vi "GoToCoordinate.vi"(0 "Target X":dbl=nan, 1 "Speed Multiplier (1)":dbl=1.0 format="%#_13g", 2 "Face PID Gains":T1={"proportional gain (Kc)"=0.275, "integral time (Ti, min)"=0.0, "derivative time (Td, min)"=0.006} {"derivative time (Td, min)" format="%.3f"; "integral time (Ti, min)" format="%.3f"; "proportional gain (Kc)" format="%.3f"}, 3 "Distance PID gains":T1={"proportional gain (Kc)"=0.0125, "integral time (Ti, min)"=0.0, "derivative time (Td, min)"=0.00225} {"derivative time (Td, min)" format="%_5g"; "integral time (Ti, min)" format="%_5g"; "proportional gain (Kc)" format="%_5g"}, 5 "Target Y":dbl=nan, 7 "Target Angle (rad)":dbl(knob)=nan scale=3.1416..-3.1416, 11 "error in (no error)":errorcluster, 12 "Position Tolerance":dbl, 14 "Angle Tolerance":dbl) -> (6 "Finished":bool, 15 "error out":errorcluster)   [LabVIEW 2015, in "Team900SwerveDrive.lvlib"]
uses:
  Team900SwerveDrive.lvlib
  SwerveGlobalData.vi
  <vilib>/addons/control/pid/NI_PID_pid.lvlib
  SwerveDriveFace.vi
  <vilib>/addons/control/pid/pid.llb/PID (DBL).vi
panel:
  out "Waveform Chart":cluster{"setpoint":dbl, dbl}(graph)
  # "Run this inside a while loop to autonomously move\nthe robot to target coordinates; the finished output\nwill become true when the robot is within tolerance\nof the target position (use this to terminate the \nwhile loop). If one or more elements of the target\ncoordinates are not wired, it will maintain the last\ninput position for that element\n\nPosition and Angle tolerance have no defaul values;\nall other terminals do not need to be wired."
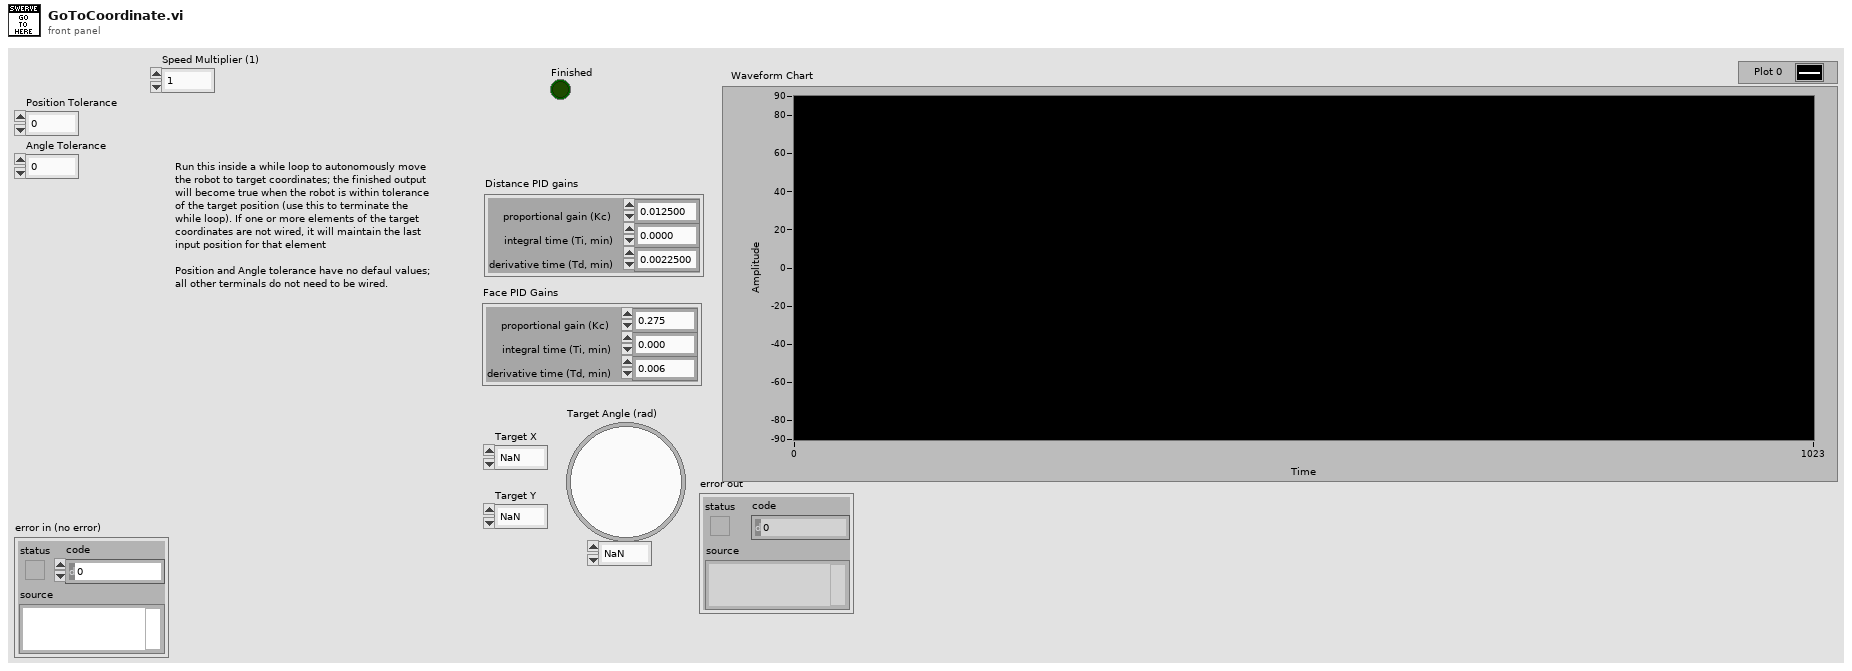
[diagram p1: front panel]
types:
  T1 = cluster{"proportional gain (Kc)":dbl, "integral time (Ti, min)":dbl, "derivative time (Td, min)":dbl}
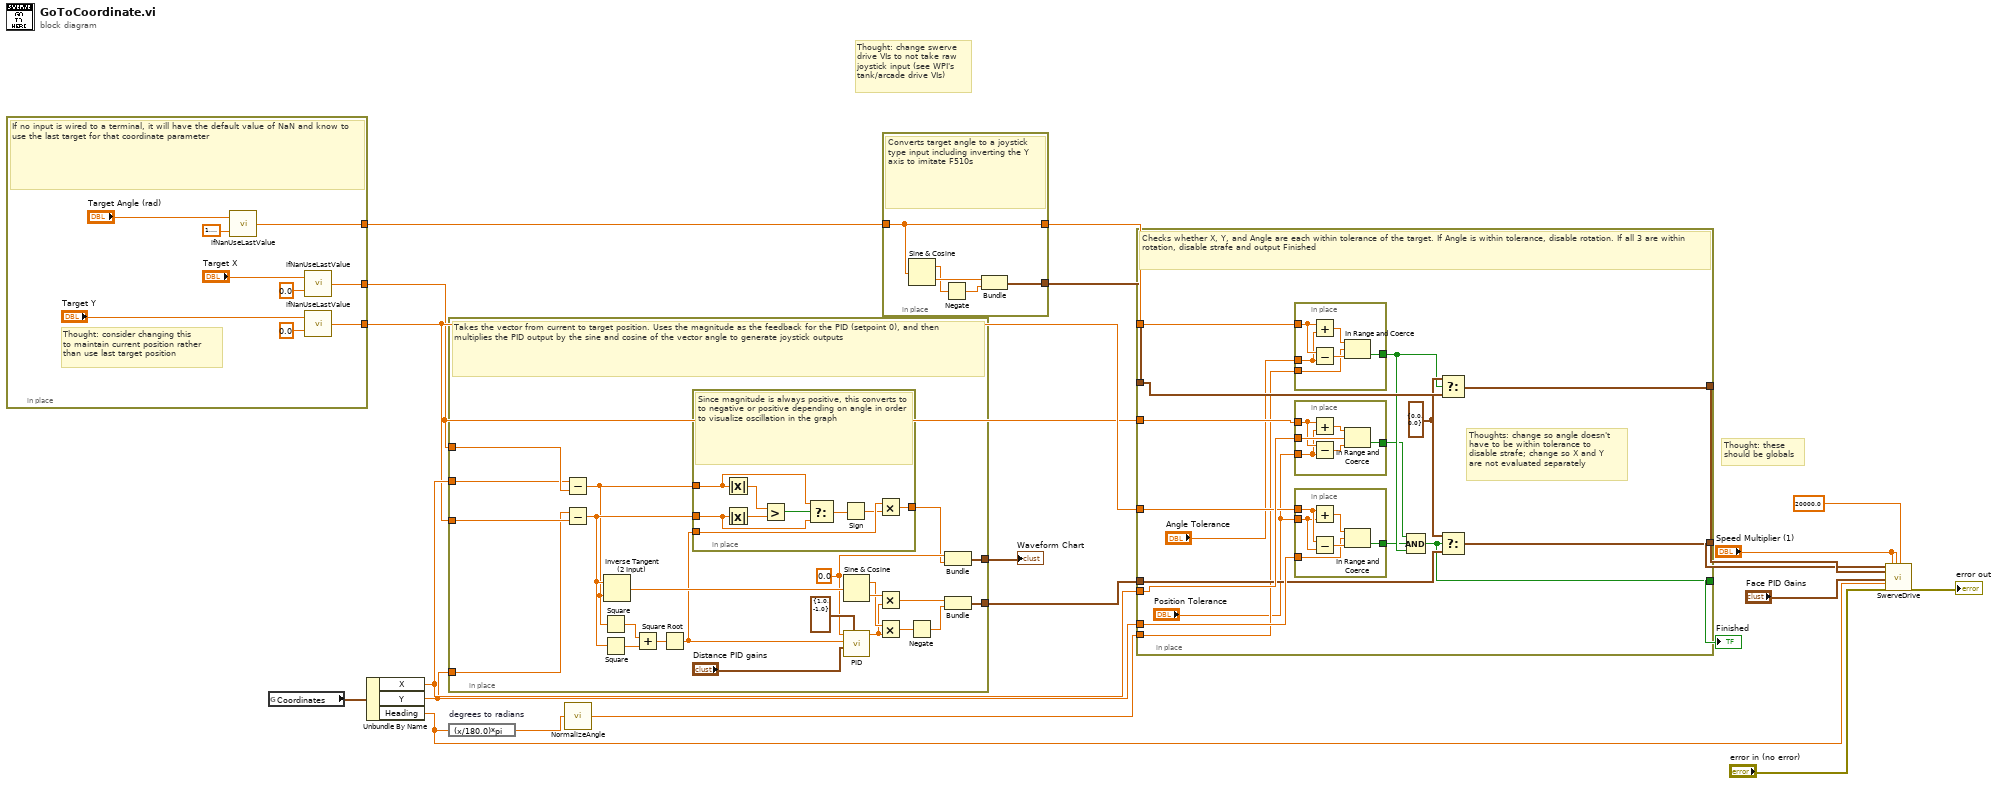
[diagram p0: block diagram]
diagram:
  # "Thought: these\nshould be globals"
  # "Thought: change swerve \ndrive VIs to not take raw \njoystick input (see WPI's\ntank/arcade drive VIs)"
  n1 = in-place {
    in-place-border: [w26] -> w5
    in-place-border: [w24] -> w4
    in-place-border: [w30] -> w6
    # "Thought: consider changing this\nto maintain current position rather \nthan use last target position"
    # "If no input is wired to a terminal, it will have the default value of NaN and know to use the last target for that coordinate parameter"
    n2 = call "ifNanUseLastValue.vi"("Starting value"=1.5707963267948966, "Number"="Target Angle (rad)") -> ("Latest num. value"=w30:dbl)
    n3 = call "ifNanUseLastValue.vi"("Starting value"=0.0, "Number"="Target X") -> ("Latest num. value"=w24:dbl)
    n4 = call "ifNanUseLastValue.vi"("Starting value"=0.0, "Number"="Target Y") -> ("Latest num. value"=w26:dbl)
  }
  n5 = global read "SwerveGlobalData.vi" "Coordinates"() -> (w18:cluster{"X":dbl, "Y":dbl, "Heading":dbl})
  n6 = Unbundle By Name(w18) -> ("X"=w17:dbl, "Y"=w16:dbl, "Heading"=w7:dbl)
  n7 = in-place {
    in-place-border: w4 -> [w45]
    in-place-border: w5 -> [w46]
    in-place-border: w17 -> [w44]
    in-place-border: w16 -> [w43]
    in-place-border: [w42] -> w9
    in-place-border: [w40] -> w12
    w39 = 0.0 ("setpoint")
    # "Takes the vector from current to target position. Uses the magnitude as the feedback for the PID (setpoint 0), and then multiplies the PID output by the sine and cosine of the vector angle to generate joystick outputs"
    n8 = Subtract(x=w44, y=w45) -> (x-y=w32:dbl)
    n9 = Subtract(x=w43, y=w46) -> (x-y=w33:dbl)
    n10 = Square(x=w32) -> (x^2=w53:dbl)
    n11 = Square(x=w33) -> (x^2=w52:dbl)
    n12 = Inverse Tangent (2 Input)(1:w32, 2:w33) -> (0:w51:dbl)
    n13 = Add(x=w53, y=w52) -> (x+y=w38:dbl)
    n14 = Square Root(x=w38) -> (sqrt(x)=w34:dbl)
    n15 = in-place {
      in-place-border: [w56] -> w35
      in-place-border: w34 -> [w62]
      in-place-border: w33 -> [w54]
      in-place-border: w32 -> [w55]
      # "Since magnitude is always positive, this converts to to negative or positive depending on angle in order to visualize oscillation in the graph"
      n16 = Absolute Value(x=w55) -> (abs(x)=w59:dbl)
      n17 = Absolute Value(x=w54) -> (abs(x)=w58:dbl)
      n18 = Greater?(x=w59, y=w58) -> (0:w57:bool)
      n19 = Select(t=w55, s=w57, f=w54) -> (s? t:f=w60:dbl)
      n20 = Sign(1:w60) -> (0:w61:dbl)
      n21 = Multiply(x=w62, y=w61) -> (x*y=w56:dbl)
    }
    n22 = Sine & Cosine(0:w51) -> (1:w49:dbl, 2:w50:dbl)
    n23 = call-poly <vilib>:"PID.vi"("output range"=cluster{"output high":dbl, "output low":dbl} {"output high"=1.0, "output low"=-1.0}, "PID gains"="Distance PID gains", "process variable"=w34, "setpoint"=w39) -> ("output"=w41:dbl)  [unwired: 6 in, 1 out]
    n24 = Multiply(x=w50, y=w41) -> (x*y=w37:dbl)
    n25 = Multiply(x=w49, y=w41) -> (x*y=w36:dbl)
    n26 = Negate(x=w36) -> (-x=w31:dbl)
    n27 = Bundle("setpoint"=w39, w35) -> (w40:cluster{"setpoint":dbl, dbl})  [unwired: 1 in]
    n28 = Bundle(w37, w31) -> (w42:cluster{dbl, dbl})  [unwired: 1 in]
  }
  "Waveform Chart" <- w12
  n29 = expression code="(x/180.0)*pi" "degrees to radians"(w7) -> (w2:dbl)
  n30 = call "NormalizeAngle.vi"("angle (rad)"=w2) -> ("angle (between pi and -pi)"=w1:dbl)
  n31 = in-place {
    in-place-border: [w67] -> w11
    in-place-border: [w66] -> w21
    in-place-border: w6 -> [w66]
    # "Converts target angle to a joystick type input including inverting the Y axis to imitate F510s"
    n32 = Sine & Cosine(0:w66) -> (1:w64:dbl, 2:w65:dbl)
    n33 = Negate(x=w64) -> (-x=w63:dbl)
    n34 = Bundle(w65, w63) -> (w67:cluster{dbl, dbl})  [unwired: 1 in]
  }
  n35 = in-place {
    in-place-border: w21 -> [w84]
    in-place-border: w17 -> [w83]
    in-place-border: w16 -> [w82]
    in-place-border: w11 -> [w81]
    in-place-border: [w80] -> w10
    in-place-border: w9 -> [w78]
    in-place-border: [w77] -> w8
    in-place-border: w5 -> [w76]
    in-place-border: w4 -> [w75]
    in-place-border: [w74] -> w3
    in-place-border: w1 -> [w72]
    w79 = cluster{dbl, dbl} {0.0, 0.0} ("t")
    # "Thoughts: change so angle doesn't\nhave to be within tolerance to\ndisable strafe; change so X and Y\nare not evaluated separately"
    # "Checks whether X, Y, and Angle are each within tolerance of the target. If Angle is within tolerance, disable rotation. If all 3 are within rotation, disable strafe and output Finished"
    n36 = in-place {
      in-place-border: [w88] -> w73
      in-place-border: w72 -> [w87]
      in-place-border: w84 -> [w86]
      in-place-border: "Angle Tolerance" -> [w85]
      n37 = Add(x=w86, y=w85) -> (x+y=w90:dbl)
      n38 = Subtract(x=w86, y=w85) -> (x-y=w89:dbl)
      n39 = In Range and Coerce(upper limit=w90, x=w87, lower limit=w89) -> (In Range?=w88:bool)  [unwired: 1 out]
    }
    n40 = in-place {
      in-place-border: [w100] -> w71
      in-place-border: w83 -> [w99]
      in-place-border: w75 -> [w98]
      in-place-border: "Position Tolerance" -> [w97]
      n41 = Add(x=w98, y=w97) -> (x+y=w102:dbl)
      n42 = Subtract(x=w98, y=w97) -> (x-y=w101:dbl)
      n43 = In Range and Coerce(upper limit=w102, x=w99, lower limit=w101) -> (In Range?=w100:bool)  [unwired: 1 out]
    }
    n44 = in-place {
      in-place-border: [w94] -> w69
      in-place-border: w82 -> [w93]
      in-place-border: w76 -> [w92]
      in-place-border: "Position Tolerance" -> [w91]
      n45 = Add(x=w92, y=w91) -> (x+y=w96:dbl)
      n46 = Subtract(x=w92, y=w91) -> (x-y=w95:dbl)
      n47 = In Range and Coerce(upper limit=w96, x=w93, lower limit=w95) -> (In Range?=w94:bool)  [unwired: 1 out]
    }
    n48 = Compound Arithmetic op=AND(w71, w69, w73) -> (w74:bool)
    n49 = Select(t=w79, s=w73, f=w81) -> (s? t:f=w80:cluster{dbl, dbl})
    n50 = Select(t=w79, s=w74, f=w78) -> (s? t:f=w77:cluster{dbl, dbl})
  }
  "Finished" <- w3
  n51 = call-poly "SwerveDrive.vi"("Strafe Joystick Axes"=w8, "Face Joystick Axes"=w10, "Face PID Gains"="Face PID Gains", "Angle (degrees; 0 = right)"=w7, "error in (no error)"="error in (no error)", "Strafe Multiplier"="Speed Multiplier (1)", "Rotation Multiplier"="Speed Multiplier (1)", "Max Wheel Speed"=20000.0) -> ("error out"=→"error out":errorcluster)  [unwired: 10 in, 1 out]
